vi "Test Default File Comparator.vi"(11 "Test Case In":refnum<class "Comparator Tests.lvclass">) -> (0 "error out":errorcluster, 3 "Test Case Out":refnum<class "Comparator Tests.lvclass">)   [LabVIEW 2020, in "Comparator Tests.lvclass"]
uses:
  Comparator Tests.lvclass
  Source/Approval Tests/File Comparator/File Comparator.lvclass
  Comparator Tests.lvclass/Comparator Tests.ctl
  C:/Program Files/National Instruments/LabVIEW 2026/vi.lib/Astemes/LUnit/Test Case.lvclass
  C:/Program Files/National Instruments/LabVIEW 2026/vi.lib/Astemes/LUnit/LUnit Runnable.lvclass
  C:/Users/SAS/Desktop/ApprovalTests.LabVIEW/Tests/Comparator Tests/Comparator Tests.lvclass
  <vilib>/Astemes/LUnit/Test Case.lvclass
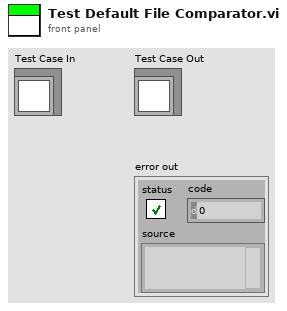
[diagram p1: front panel]
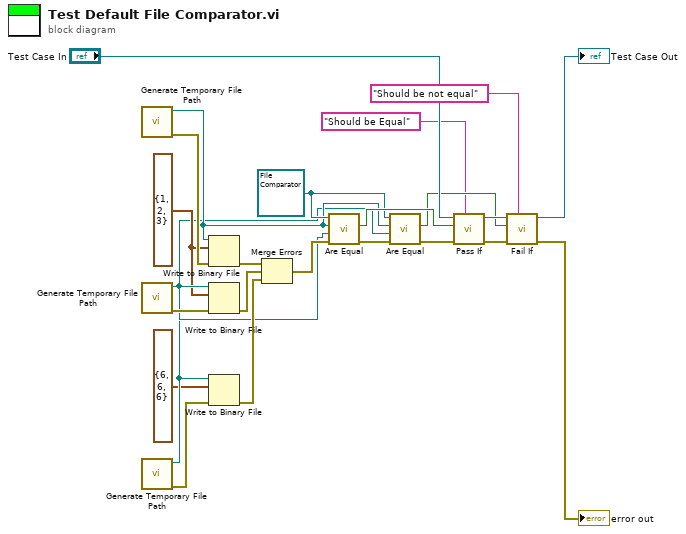
[diagram p0: block diagram]
diagram:
  w6 = cluster{"A":i32, "B":i32, "C":i32} {"A"=1, "B"=2, "C"=3}
  w9 = refnum<class "File Comparator.lvclass"> refnum ("Approval Tests:File Comparator.lvclass")
  n1 = call <vilib>:"Generate Temporary File Path.vi"() -> ("error out"=w22:errorcluster, "Unique Temporary File Path"=w5:path)  [unwired: 10 in]
  n2 = call <vilib>:"Generate Temporary File Path.vi"() -> ("error out"=w21:errorcluster, "Unique Temporary File Path"=w7:path)  [unwired: 10 in]
  n3 = call <vilib>:"Generate Temporary File Path.vi"() -> ("error out"=w20:errorcluster, "Unique Temporary File Path"=w4:path)  [unwired: 10 in]
  n4 = Write to Binary File(file (use dialog)=w5, data=w6, error in=w22) -> (error out=w19:errorcluster)  [unwired: 3 in, 2 out]
  n5 = Write to Binary File(file (use dialog)=w7, data=w6, error in=w21) -> (error out=w18:errorcluster)  [unwired: 3 in, 2 out]
  n6 = Write to Binary File(file (use dialog)=w4, data=cluster{"A":i32, "B":i32, "C":i32} {"A"=6, "B"=6, "C"=6}, error in=w20) -> (error out=w17:errorcluster)  [unwired: 3 in, 2 out]
  n7 = Merge Errors(w19, w18, w17) -> (w16:errorcluster)
  n8 = call-dynamic "Are Equal.vi"("error in"=w16, "Recieved File Path"=w7, "Approved File Path"=w5, "File Comparator in"=w9) -> ("error out"=w15:errorcluster, "Are Equal?"=w12:bool)  [unwired: 5 in, 1 out]
  n9 = call-dynamic "Are Equal.vi"("error in"=w15, "Recieved File Path"=w4, "Approved File Path"=w5, "File Comparator in"=w9) -> ("error out"=w14:errorcluster, "Are Equal?"=w8:bool)  [unwired: 5 in, 1 out]
  n10 = call <vilib>:"Pass If.vi"("Description"="Should be Equal", "error in (no error)"=w14, "Pass?"=w12, "LUnit Test Case In"="Test Case In") -> ("error out"=w24:errorcluster, "LUnit Test Case Out"=w11:refnum<class "Comparator Tests.lvclass">)  [unwired: 6 in]
  n11 = call <vilib>:"Fail If.vi"("Description"="Should be not equal", "error in (no error)"=w24, "Fail?"=w8, "LUnit Test Case In"=w11) -> ("error out"=→"error out":errorcluster, "LUnit Test Case Out"=→"Test Case Out":refnum<class "Comparator Tests.lvclass">)  [unwired: 6 in]
